vi "CRYMisc vis settings global.vi"() -> ()   [LabVIEW 2013]
uses:
  Typedef Control/CRYScope-FFT.ctl
  Typedef Control/CRYMultimeter.ctl
panel:
  in  "Rcv Index Array":T1(array[cluster])
  in  "Main Rcv":i32[](array[numeric])=[-1, -1, -1, -1, -1, -1, -1, -1, -1, -1, -1, -1, -1, -1, -1]
  in  "Main Gen":i32[](array[numeric])=[-1, -1, -1, -1, -1, -1, -1, -1, -1, -1, -1, -1, -1, -1, -1]
  in  "Generator Index Array":T2(array[cluster])
  in  "g_OpenedChannels":T3(array[cluster])
  in  "g_OpendAsioDev":cluster{"Dev Name":string, "Count":i16}
  in  "Operator Start File":path
  in  "OpenAll Event":bool
  in  "Operator Work Path":path
  in  "CloseAll Event":bool
  in  "gOperator Msg VI Ref":refnum<vi>
  in  "CloseAll":bool
  out "Temp VI nID":i32
  out "Temp Title nID":i32
  out "RTA":T4
  out "Oscillo":T4
  out "Multimeter":T4
  out "SigGen":T4
  in  "scope-fft mode":u32(ring)=1 items=["Time", "Spectrum"]
  in  "Menu?":bool
  in  "Manual":bool
  in  "Mute":bool
  out "Execution control":T5
  out "Voltmeter Settings":T6={"Ave/Max/Min"=0, "Level"=0, "Channel"=0, "Signal Type"="None", "Weighting"="None", "Applay Correction"=FALSE, "lin/exp avg"=0, "rec time (sec)"=0.0009999999999998899, "Average Time (Sec)"=0.0009999999999998899, "Lin Display Prefs"="%#_6p", "dB Display Prefs"="%.1f", "Time Weighting"=0, "Display"=0}
  in  "Scope-FFT settings":T7={"window"=0, "n avgs"=1, "lin/exp avg"=0, "pwr/cplx avg"=0, "time (ms)"=0.0, "fft lines"=2048, "scope/fft mode"=0, "channel"=0, "trig. channel"=0, "Applay Correction"=FALSE, "Time Display"="%#_6p", "Freq. Weighting"="%.1f", "Ave/Max/Min"=0, "Trigger Level"=0.0, "Trigger Unit"=2, "Trigger Time Offset"=0.0, "Trigger Slope"=0, "Trigger/Free Run"=FALSE, "continuous"=FALSE, "Spectrum Display"="%#_6p", "Calc FFT"=FALSE, "Y-axis"="None", "Signal Type"=""} {"Trigger Time Offset" format="%.2f"; "Trigger Level" format="%.2f"; "time (ms)" format="%.2f"}
  in  "RTA settings":T8 {"det sec" format="%.2f"}
  in  "Signal Gen'r settings":T9={"gen'r mode"=0, "frequency"=0, "output level"=0.0, "wave path"="", "wav play mode"=0, "duration"=0.0, "n times"=0, "channel"=0, "wav level"=0.0, "EQ"=FALSE, "f knob log"=FALSE, "f knob low"=0.0, "f knob high"=0.0, "ol knob log"=FALSE, "ol knob low"=0.0, "ol knob high"=0.0, "Lin Display Prefs"="%#_6p", "dB Display Prefs"="%.1f", "Duration noise"=20.0, "Min freq noise"=20.0, "Max freq noise"=20000.0, "Signal Type"="", "Play Sine Wave"=0} {"Duration noise" format="%.2f"; "Max freq noise" format="%.2f"; "Min freq noise" format="%.2f"; "ol knob high" format="%.2f"; "ol knob low" format="%.2f"; "f knob high" format="%.2f"; "f knob low" format="%.2f"; "wav level" format="%.2f"; "duration" format="%.2f"; "output level" format="%.2f"}
  # "Operator"
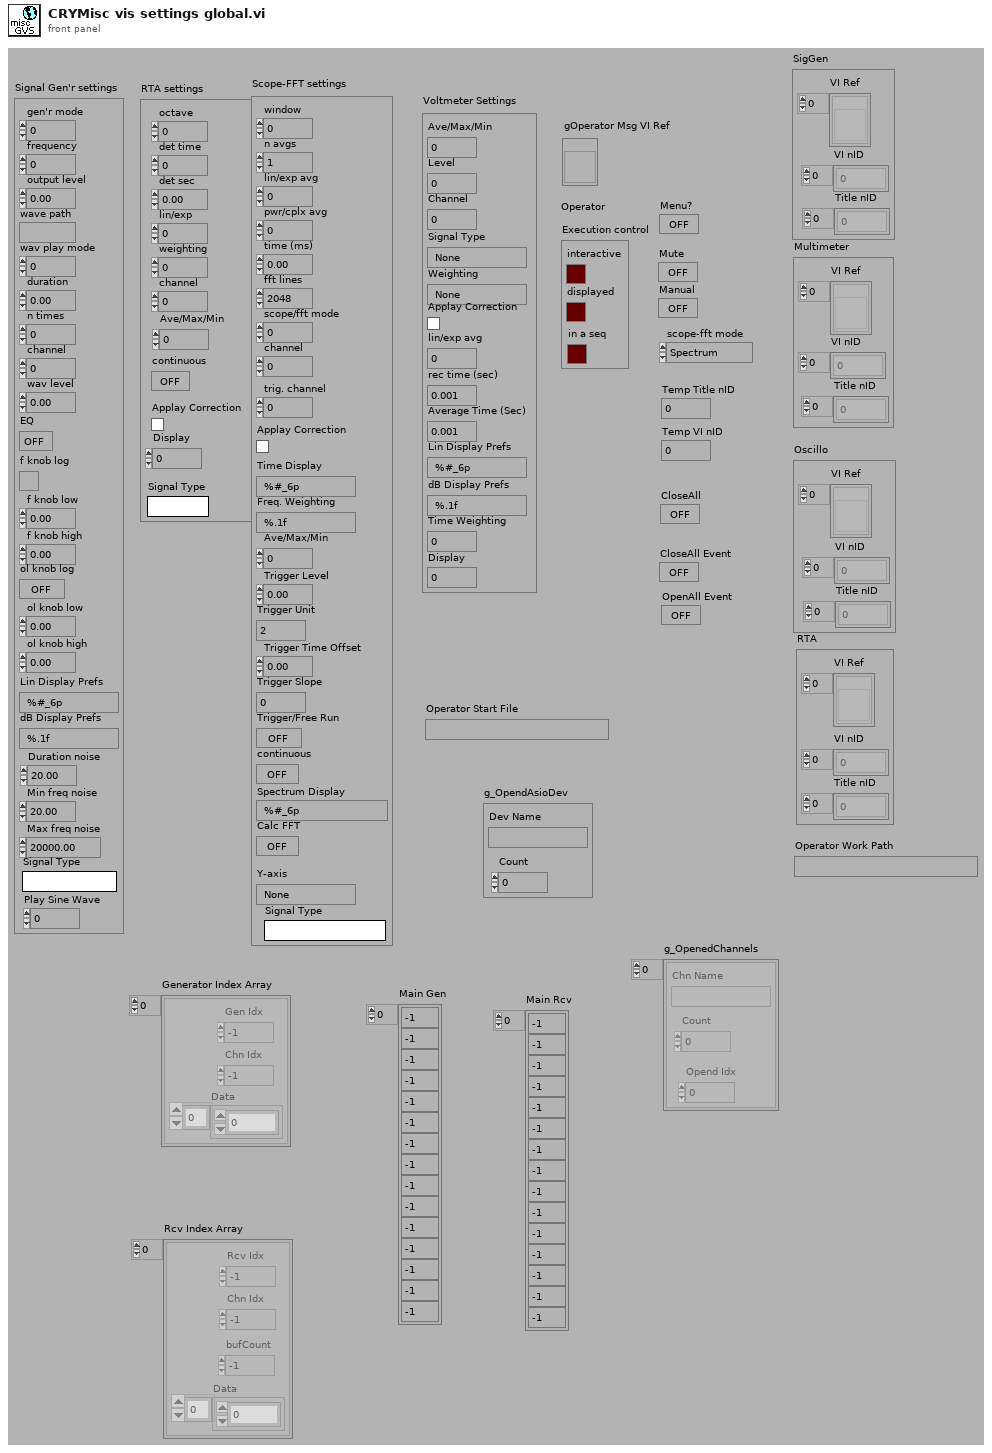
[diagram p1: front panel]
types:
  T1 = cluster{"Rcv Idx":i32, "Chn Idx":i32, "Data":i32[], "bufCount":i32}[]
  T2 = cluster{"Gen Idx":i32, "Chn Idx":i32, "Data":sgl[]}[]
  T3 = cluster{"Chn Name":string, "Count":i16, "Opend Idx":i16}[]
  T4 = cluster{"VI Ref":refnum<vi>[], "VI nID":i32[], "Title nID":i32[]}
  T5 = cluster{"interactive":bool, "displayed":bool, "in a seq":bool}
  T6 = typedef "CRYMultimeter.ctl" = cluster{"Ave/Max/Min":i32, "Level":i32, "Channel":i32, "Signal Type":string, "Weighting":string, "Applay Correction":bool, "lin/exp avg":u16, "rec time (sec)":dbl, "Average Time (Sec)":dbl, "Lin Display Prefs":string, "dB Display Prefs":string, "Time Weighting":u16, "Display":u16}
  T7 = typedef "CRYScope-FFT.ctl" = cluster{"window":i32, "n avgs":i32, "lin/exp avg":i32, "pwr/cplx avg":i32, "time (ms)":dbl, "fft lines":i32, "scope/fft mode":i32, "channel":i32, "trig. channel":i32, "Applay Correction":bool, "Time Display":string, "Freq. Weighting":string, "Ave/Max/Min":u16, "Trigger Level":dbl, "Trigger Unit":u16, "Trigger Time Offset":dbl, "Trigger Slope":u16, "Trigger/Free Run":bool, "continuous":bool, "Spectrum Display":string, "Calc FFT":bool, "Y-axis":string, "Signal Type":string}
  T8 = cluster{"octave":i32, "det time":i32, "det sec":dbl, "lin/exp":i32, "weighting":i32, "channel":i32, "Ave/Max/Min":u16, "continuous":bool, "Applay Correction":bool, "Display":u16, "Signal Type":string}
  T9 = cluster{"gen'r mode":i32, "frequency":u32, "output level":dbl, "wave path":string, "wav play mode":i32, "duration":dbl, "n times":i32, "channel":i32, "wav level":dbl, "EQ":bool, "f knob log":bool, "f knob low":dbl, "f knob high":dbl, "ol knob log":bool, "ol knob low":dbl, "ol knob high":dbl, "Lin Display Prefs":string, "dB Display Prefs":string, "Duration noise":dbl, "Min freq noise":dbl, "Max freq noise":dbl, "Signal Type":string, "Play Sine Wave":i32}
diagram:
